vi "writeRS232.vi"(8 "error in (no error)":errorcluster, 9 "Data":u8[](array[numeric]), 10 "Port":u8, 11 "FPGA in":refnum<class "FPGA.lvclass">) -> (0 "error out":errorcluster, 3 "FPGA out":refnum<class "FPGA.lvclass">)   [LabVIEW 2016, in "FPGA.lvclass"]
uses:
  FPGA.lvclass
  FPGA.lvclass/FPGA.ctl
  <vilib>/Utility/error.llb/Error Cluster From Error Code.vi
  <vilib>/rvi/errors/niLvFpgaAdjustHostInterfaceError.vi
  <vilib>/rvi/interface/nirviMethod/nirviMethod.xnode
  <vilib>/FPGAPlugInAG/Dynamic/niLvFpga_WriteFifo_Dynamic.vi
  <vilib>/rvi/errors/niLvFpgaMergeErrorWithErrorCode.vi
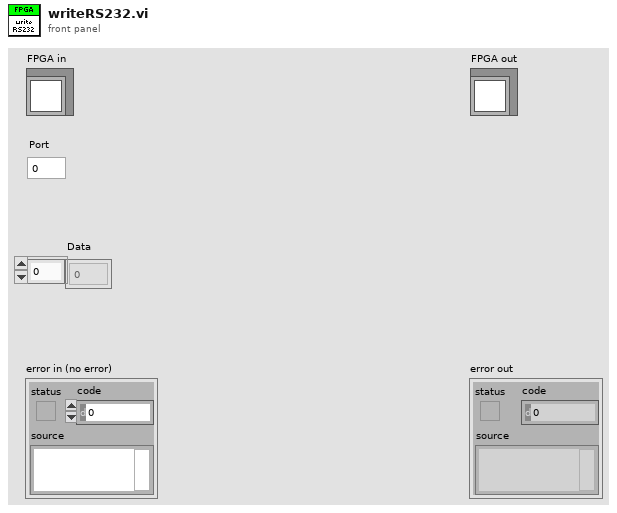
[diagram p1: front panel]
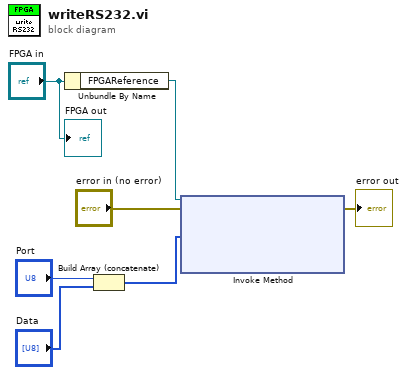
[diagram p0: block diagram]
diagram:
  n1 = Unbundle By Name("FPGA in") -> ("FPGAReference"=w6:refnum<k20>)
  n2 = Build Array (concatenate)("Port", "Data") -> (w1:u8[])
  n3 = xnode "Invoke Method"("FPGA VI Reference In"=w6, "error in"="error in (no error)", "Data"=w1) -> ("error out"=→"error out":errorcluster)  [unwired: 1 in, 2 out]
  "FPGA out" <- "FPGA in"
